vi "Convert To Little Endian Byte Array (U32).vi"(1 "Value":u32) -> (0 "Byte Array":u8[](array[numeric]))   [LabVIEW 2020]
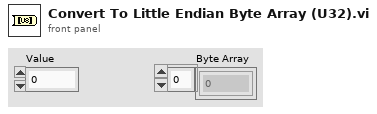
[diagram p1: front panel]
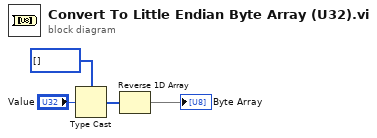
[diagram p0: block diagram]
diagram:
  n1 = Type Cast(type=u8[] [] ("Array in"), x="Value") -> (*(type *) &x=w2:u8[])
  n2 = Reverse 1D Array(array=w2) -> (reversed array=→"Byte Array":u8[])
